vi "About program (SubVI).vi"(10 "Application Directory":path, 11 "EC_About_prg in":T1) -> (2 "String":string, 3 "EC_About_prg out":T1)   [LabVIEW 2017]
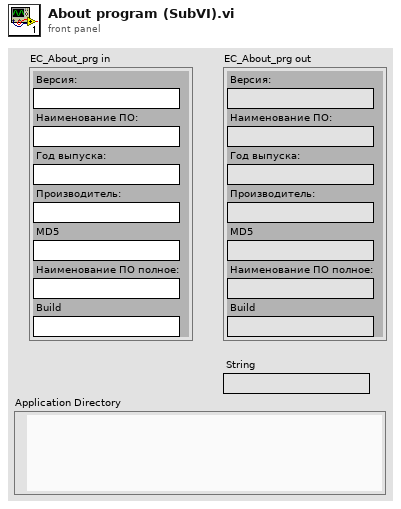
[diagram p1: front panel]
types:
  T1 = cluster{"Версия:":string, "Наименование ПО:":string, "Год выпуска:":string, "Производитель:":string, "MD5":string, "Наименование ПО полное:":string, "Build":string}
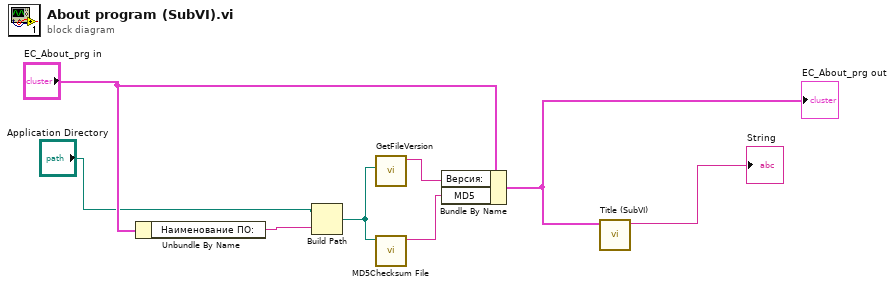
[diagram p0: block diagram]
diagram:
  n1 = Unbundle By Name("EC_About_prg in") -> ("Наименование ПО:"=w6:string)
  n2 = Build Path(base path="Application Directory", name or relative path=w6) -> (appended path=w7:path)
  n3 = call "GetFileVersion.vi"("path"=w7) -> ("Full version"=w4:string)  [unwired: 10 in]
  n4 = call <vilib>:"MD5Checksum File.vi"("Path"=w7) -> ("MD5 message-digest"=w8:string)  [unwired: 9 in, 1 out]
  n5 = Bundle By Name(cluster="EC_About_prg in", "Версия:"=w4, "MD5"=w8) -> (w2:T1)
  "EC_About_prg out" <- w2
  n6 = call "Title (SubVI).vi"("About_prg"=w2) -> ("String"=→"String":string)  [unwired: 10 in]
